vi "FGV Queue.vi"(8 "error in (no error)":errorcluster, 10 "FGV Queue State":T1, 11 "queue in":refnum<queue>) -> (0 "error out":errorcluster, 3 "queue out":refnum<queue>)   [LabVIEW 2023, in "Template.lvlib"]
doc: "VI used to store queue ref to be used in the module."
uses:
  Template.lvlib
  Type Def/FGV Queue State.ctl
  Type Def/Message Data.ctl
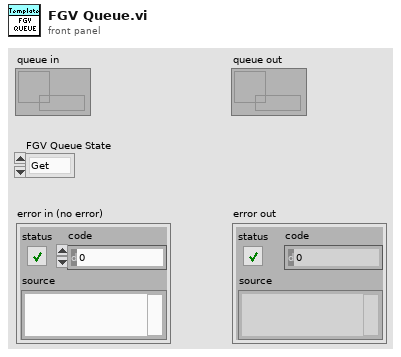
[diagram p1: front panel]
types:
  T1 = typedef "Template.lvlib/FGV Queue State.ctl" = enum16{"Get", "Set"}
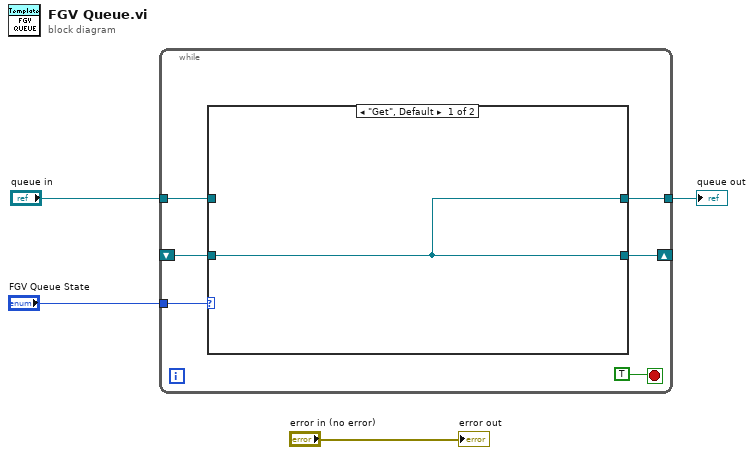
[diagram p0: block diagram]
diagram:
  n1 = while {
    tunnel: "FGV Queue State" -> [w10]
    tunnel: "queue in" -> [w8]
    tunnel: [w7] -> w1
    shift-right: [w6] -> _
    shift-left: _ -> [w5]
    stop <- TRUE stop-if-true
    n2 = case shown="\"Get\", Default" w10 {
      tunnel: w8 -> [_ w12]
      tunnel: [w11 w12] -> w7
      tunnel: [w11 w12] -> w6
      tunnel: w5 -> [w11 _]
      frame "Get", Default {
      }
      frame "Set" {
      }
    }
  }
  "queue out" <- w1
  "error out" <- "error in (no error)"
